vi "OAT Polar Draw Orbit Plot.vi"(0 "picture":picture, 1 "polar settings":T3={"polar attributes"={"maximum"=2.0, "minimum"=0.0, "clip to min"=FALSE, "log"=FALSE, "grid color"=3381657, "plot color"=16711680, "fmt and prec"={"format"=enum."Decimal", "precision"=2}, "visible section"=4}, "desired font"=enum."Application Font", "user-specified font"={"Font Name:"="", "Size"=0, "Strikeout?"=FALSE, "Italic?"=FALSE, "Underline?"=FALSE, "Outline?"=FALSE, "Shadow?"=FALSE, "Bold?"=FALSE}} {"polar attributes"."minimum" format="%.2f"; "polar attributes"."maximum" format="%.2f"}, 2 "Cursor List (EU position]":T2(array[cluster]) {"Location"."phase" format="%.2f"; "Location"."mag" format="%.2f"}, 3 "cursor attributes":T4={"layout color"=852223, "active color"=16740820, "precision"=2, "BG transparent? (T)"=FALSE, "radius"=2}, 5 "magnitudes (even angular)":dbl[](array[numeric]) format="%.2f", 7 "phases":dbl[](array[numeric]) format="%.2f", 9 "picture \ndimensions (w,h)":cluster{"width":i16, "height":i16}, 12 "channel settings":T1 {"probe angle [deg]" max=360 step=1; "shaft rotating direction" items=["CCW", "CW"]}, 14 "avoid overlap? (Y)":bool=TRUE) -> (4 "picture out":picture, 6 "grid measurements out":T5 {"end angle" format="%.2f"; "start angle" format="%.2f"; "scale factors"."b" format="%.2f"; "scale factors"."a" format="%.2f"})   [LabVIEW 2017]
uses:
  <vilib>/addons/Sound and Vibration/Order Analysis/Backward Compatibility/SubVIs/OAT Polar Cursor Attributes.ctl
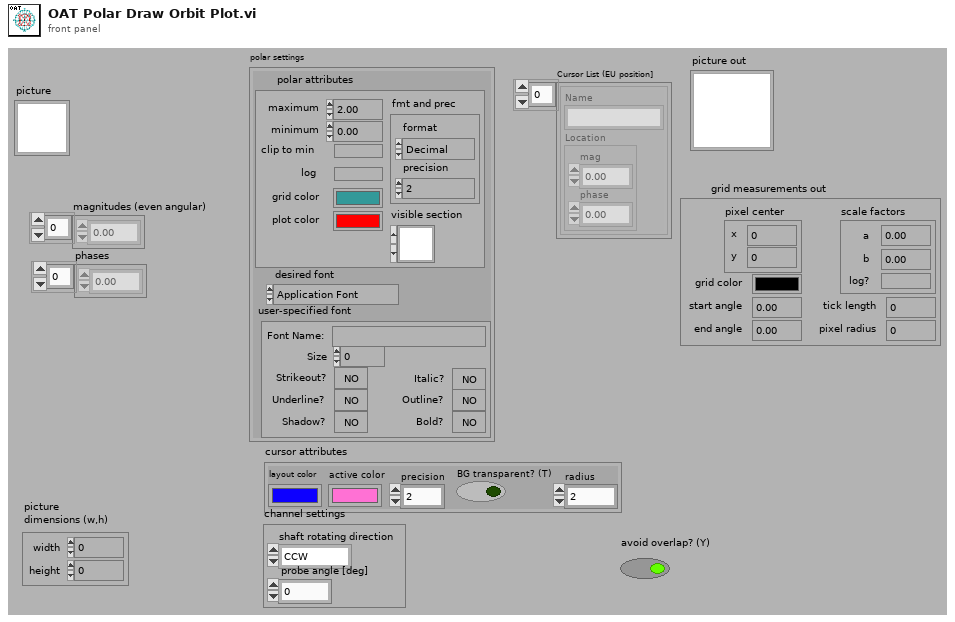
[diagram p1: front panel]
types:
  T1 = cluster{"shaft rotating direction":u16, "probe angle [deg]":u16}
  T2 = cluster{"Name":string, "Location":cluster{"mag":dbl, "phase":dbl}}[]
  T3 = cluster{"polar attributes":cluster{"maximum":dbl, "minimum":dbl, "clip to min":bool, "log":bool, "grid color":u32, "plot color":u32, "fmt and prec":cluster{"format":enum8{"Decimal", "Scientific", "Engineering", "Binary", "Octal", "Hex"}, "precision":u8}, "visible section":u16}, "desired font":enum16{"User-specified Font", "Application Font", "System Font", "Dialog Font"}, "user-specified font":cluster{"Font Name:":string, "Size":i16, "Strikeout?":bool, "Italic?":bool, "Underline?":bool, "Outline?":bool, "Shadow?":bool, "Bold?":bool}}
  T4 = typedef "OAT Polar Cursor Attributes.ctl" = cluster{"layout color":u32, "active color":u32, "precision":i16, "BG transparent? (T)":bool, "radius":i16}
  T5 = cluster{"pixel center":cluster{"x":i16, "y":i16}, "scale factors":cluster{"a":dbl, "b":dbl, "log?":bool}, "grid color":u32, "start angle":dbl, "end angle":dbl, "tick length":i16, "pixel radius":i32}
  T6 = cluster{"line color":u32, "text color":u32, "tick length(3)":i16, "crossing axes":bool, "visible grid?":bool}
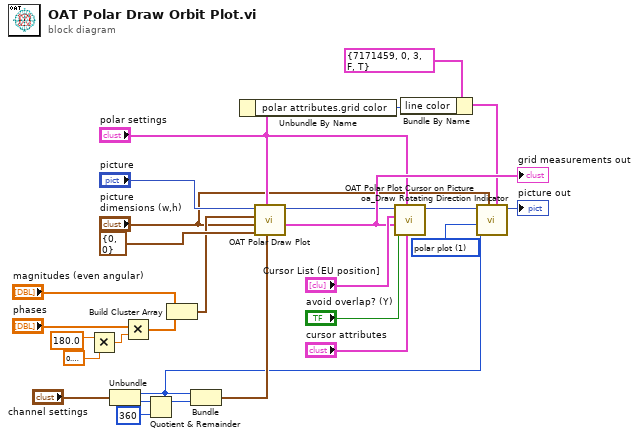
[diagram p0: block diagram]
diagram:
  w1 = u16 1 items=["shaft centerline plot", "polar plot"] ("plot type")
  n1 = Multiply(x=180.0, y=0.3183098861837907) -> (x*y=w23:dbl)
  n2 = Unbundle("channel settings") -> ("shaft rotating direction"=w8:u16, "probe angle [deg]"=w13:u16)
  n3 = Multiply(x="phases", y=w23) -> (x*y=w20:dbl[])
  n4 = Quotient & Remainder(x=w13, y=u16 360) -> (x-y*floor(x/y)=w11:u16)  [unwired: 1 out]
  n5 = Build Cluster Array("magnitudes (even angular)", w20) -> (w19:cluster{dbl, dbl}[])
  n6 = Bundle("shaft rotating direction"=w8, w11) -> (w10:cluster{"shaft rotating direction":u16, u16})  [unwired: 1 in]
  n7 = Unbundle By Name("polar settings") -> ("polar attributes.grid color"=w4:u32)
  n8 = call <vilib>:"OAT Polar Draw Plot.vi"("channel settings"=w10, "polar settings"="polar settings", "top left point(0, 0)"=cluster{"x":i16, "y":i16} {"x"=0, "y"=0}, "dimensions (w,h)"="picture \ndimensions (w,h)", "data array [mag, phase (deg)]"=w19, "picture"="picture") -> ("grid measurements"=w16:T5, "new picture"=w15:picture)  [unwired: 4 in]
  "grid measurements out" <- w16
  n9 = call <vilib>:"OAT Polar Plot Cursor on Picture.vi"("cursor attributes"="cursor attributes", "polar settings"="polar settings", "avoid overlap? (Y)"="avoid overlap? (Y)", "grid measurements in"=w16, "Cursor List"="Cursor List (EU position]", "picture"=w15) -> ("new picture"=w9:picture)  [unwired: 4 in, 1 out]
  n10 = Bundle By Name(cluster=T6 {"line color"=7171459, "text color"=0, "tick length(3)"=3, "crossing axes"=FALSE, "visible grid?"=TRUE} ("cartesian grid cosmetics"), "line color"=w4) -> (w3:T6)
  n11 = call <vilib>:"oa_Draw Rotating Direction Indicator.vi"("cartesian grid cosmetics"=w3, "picture \ndimensions (w,h)"="picture \ndimensions (w,h)", "shaft rotating direction"=w8, "plot type"=w1, "picture"=w9) -> ("new picture"=→"picture out":picture)  [unwired: 6 in]
